vi "AlliGator Shot Noise Influence on Average Lifetime.vi"() -> ()   [LabVIEW 2021, in "AlliGator Shot Noise Influence on Average Lifetime.lvlib"]
doc: "Main window of the Shot Noise Influence on Average Lifetime tool."
uses:
  AlliGator Shot Noise Influence on Average Lifetime.lvlib
  AlliGator Statistics Simulation Parameters.ctl
  AlliGator Phasor Simulation Parameters.ctl
  Arrays/Array Statistics.ctl
  Graphs/XY Graph/XY Graph Event.ctl
  <vilib>/Utility/miscctls.llb/LVPoint32TypeDef.ctl
  1e2fc33e-f2e1-4865-bd35-b782600da79c.vi
  ffbda573-fdee-4728-9e4a-091745fb94a5.vi
  20485d49-49ee-422f-9a66-761cdf75a503.vi
  AlliGator Abort.vi
  GUI/GUI.lvlib
  Notebook/Notebook.lvlib
  Error/Error.lvlib
  AlliGator Globals, Variables & Constants.lvlib
  Graphs/XY Graph/XY Graph Add-Ons.lvlib
  Arrays/Arrays.lvlib
panel:
  in  "Random Seed":i32=1000
  in  "SDV Histogram Percentiles":dbl[](array[numeric])=[1.0, 99.0]
  in  "Lifetime Histogram Percentiles":dbl[](array[numeric])=[1.0, 99.0]
  out "Message":string caption="Output (see Notebook)"
  in  "Histogram Bin Size (SDV)":dbl[unit]=1.0000000000000002e-12
  out "AlliGator Approach SDVs":T1 {"Min" format="%#_4g"; "Max" format="%#_4g"; "Mean" format="%#_4g"; "Standard Deviation" format="%#_4g"}
  out "AlliGator Approach":T1 {"Min" format="%#_4g"; "Max" format="%#_4g"; "Mean" format="%#_4g"; "Standard Deviation" format="%#_4g"}
  out "Pure Poisson":T1 {"Min" format="%#_4g"; "Max" format="%#_4g"; "Mean" format="%#_4g"; "Standard Deviation" format="%#_4g"}
  in  "Histogram Bin Size (Lifetime)":dbl[unit]=1.0000000000000001e-11
  in  "Phasor Parameters":T2={"tau 1"=3e-10, "tau 2"=3.0000000000000004e-09, "f1"=0.5, "Frequency"=80000000.0}
  in  "Simulation Parameters":T3={"# Photons"=100, "# Replicas (M)"=1000, "# Simulations (N)"=1000, "Decay Bin Size"=1.0000000000000002e-10}
  in  "Run Simulation":bool
  out "Histograms":cluster{"Axis":dbl[], "Histogram":dbl[]}[](graph)
  in  "Animated Busy Icon":bool=TRUE
  in  "Abort":bool
  out "Progress Bar":dbl(slide) scale=0.0..100.0
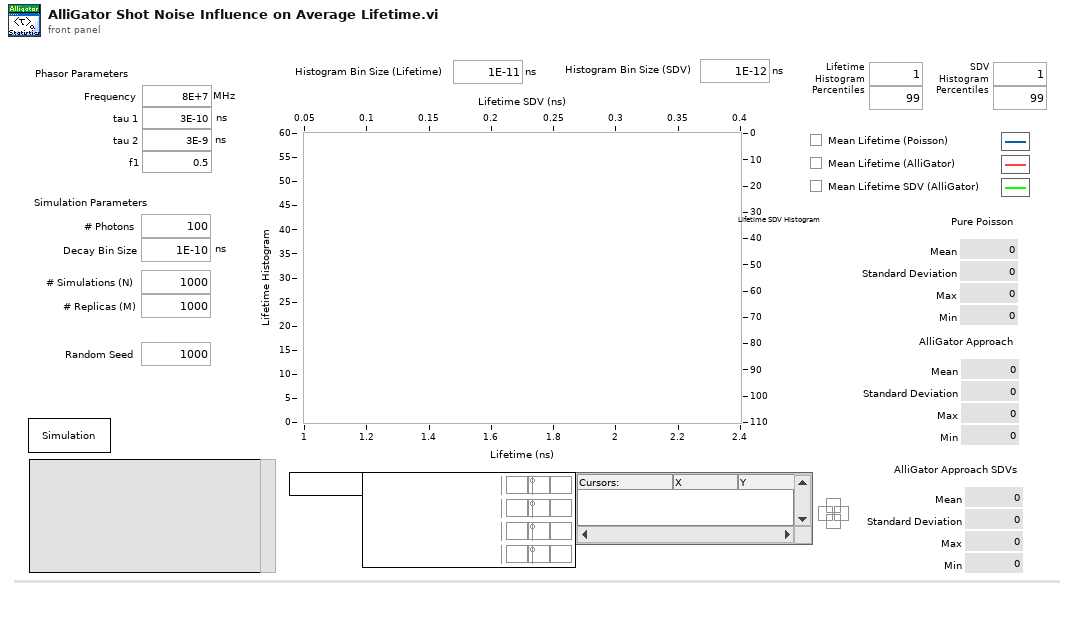
[diagram p1: front panel]
types:
  T1 = typedef "Arrays.lvlib/Array Statistics.ctl" = cluster{"Mean":dbl, "Standard Deviation":dbl, "Max":dbl, "Min":dbl}
  T2 = typedef "AlliGator Shot Noise Influence on Average Lifetime.lvlib/AlliGator Phasor Simulation Parameters.ctl" = cluster{"tau 1":dbl[unit], "tau 2":dbl[unit], "f1":dbl, "Frequency":dbl[unit]}
  T3 = typedef "AlliGator Shot Noise Influence on Average Lifetime.lvlib/AlliGator Statistics Simulation Parameters.ctl" = cluster{"# Photons":i32, "# Replicas (M)":i32, "# Simulations (N)":i32, "Decay Bin Size":dbl[unit]}
  T4 = typedef "XY Graph Add-Ons.lvlib/XY Graph Event.ctl" = cluster{"Item Tag":string, "XY Graph Refnum":refnum<vi>, "Coords":T5, "Item Path":string}
  T5 = typedef "LVPoint32TypeDef.ctl" = cluster{"Horizontal":i32, "Vertical":i32}
  T6 = typedef "AlliGator Progress Bar Q Element.ctl" = cluster{"Action":string, "Value":dbl}
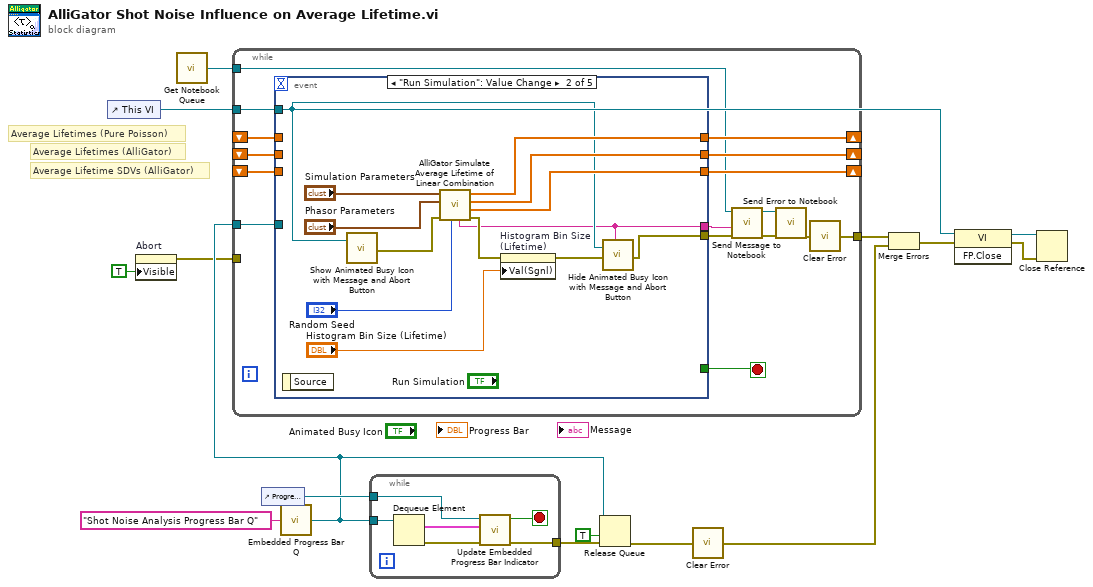
[diagram p0: block diagram]
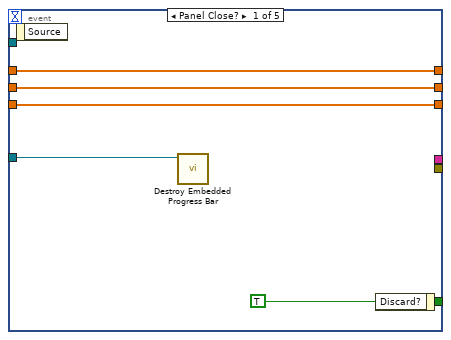
[diagram p2: hidden frame]
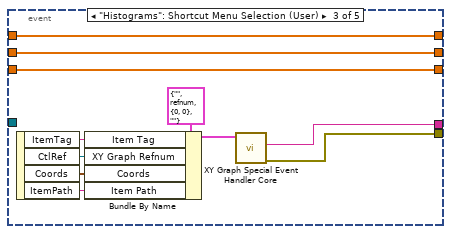
[diagram p3: hidden frame]
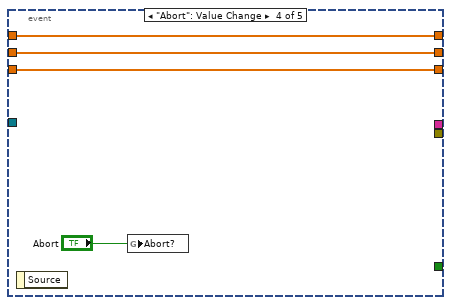
[diagram p4: hidden frame]
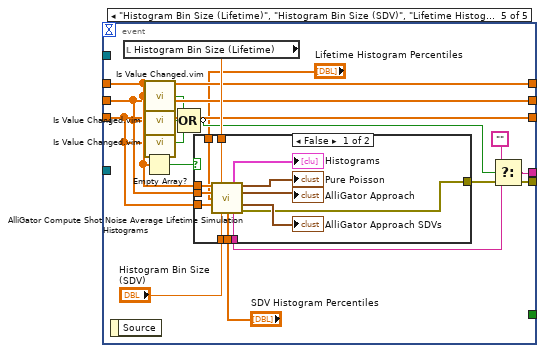
[diagram p5: hidden frame]
diagram:
  # "Average Lifetime SDVs (AlliGator)"
  # "Average Lifetimes (AlliGator)"
  # "Average Lifetimes (Pure Poisson)"
  n1 = control-ref of="This VI"() -> (w2:refnum<vi>)
  n2 = property on="Abort" class="Bool"("Visible"=TRUE) -> (error out=w3:errorcluster)  [unwired: 2 in, 1 out]
  n3 = call "Get Notebook Queue.vi"() -> ("Notebook Queue"=w10:refnum<queue>)  [unwired: 9 in]
  n4 = control-ref of="Progress Bar"() -> (w14:refnum<vi>)
  n5 = call "Embedded Progress Bar Q.vi"("Progress Bar Queue Name"="Shot Noise Analysis Progress Bar Q") -> ("Progress Bar Queue"=w11:refnum<queue>)  [unwired: 6 in]
  n6 = while {
    shift-right: [w30] -> _
    shift-left: _ -> [w27]
    shift-right: [w29] -> _
    shift-left: _ -> [w26]
    shift-right: [w28] -> _
    shift-left: _ -> [w25]
    tunnel: w11 -> [w24]
    tunnel: w10 -> [w23]
    tunnel: [w17] -> w9
    tunnel: w3 -> [_]
    tunnel: w2 -> [w16]
    stop <- w31 stop-if-true
    n7 = event shown="[1] \"Run Simulation\": Value Change" {
      selector: _ -> [_ _ _ _ _]
      dyn-events: _ -> [_ _ _ _ _]
      timeout: _ -> [_ _ _ _ _]
      tunnel: [w36 _ _ _ _] -> w31
      tunnel: [w35 w47 w60 w64 w76] -> w30
      tunnel: [w34 w46 w59 w63 w75] -> w29
      tunnel: [w33 w45 w58 w62 w74] -> w28
      tunnel: w27 -> [w35 _ w60 w64 w76]
      tunnel: w26 -> [w34 _ w59 w63 w75]
      tunnel: w25 -> [w33 _ w58 w62 w74]
      tunnel: w24 -> [w32 _ _ _ _]
      tunnel: [_ w38 w51 _ w68] -> w22
      tunnel: [_ w40 w50 _ w78] -> w18
      tunnel: w16 -> [_ w39 _ _ _]
      event Panel Close? {
        w36 = TRUE ("Discard?")
        n8 = event-data() -> ()  [unwired: 1 in, 1 out]
        n9 = call "Destroy Embedded Progress Bar.vi"("Progress Bar Queue in"=w32) -> ()  [unwired: 10 in, 1 out]
        n10 = event-data("Discard?"=w36) -> ()  [unwired: 1 in, 1 out]
      }
      event "Run Simulation": Value Change {
        n11 = event-data() -> ()  [unwired: 1 in, 1 out]
        n12 = call "Show Animated Busy Icon with Message and Abort Button.vi"("Target VI reference"=w39) -> ("Error Out"=w42:errorcluster)  [unwired: 18 in]
        n13 = call "AlliGator Simulate Average Lifetime of Linear Combination.vi"("seed"="Random Seed", "Error In"=w42, "Phasor Parameters"="Phasor Parameters", "Simulation Parameters"="Simulation Parameters") -> ("Error Out"=w43:errorcluster, "Average Lifetimes SDV (AlliGator)"=w45:dbl[], "Average Lifetimes (AlliGator)"=w46:dbl[], "Average Lifetimes (Pure Poisson)"=w47:dbl[], "Message"=w38:string)  [unwired: 3 in]
        n14 = property on="Histogram Bin Size (Lifetime)" class="DigNum (strict)"(error in=w43, "Val(Sgnl)"="Histogram Bin Size (Lifetime)") -> (error out=w41:errorcluster)  [unwired: 1 in, 1 out]
        n15 = call "Hide Animated Busy Icon with Message and Abort Button.vi"("Message"=w38, "Target VI reference"=w39, "Error In"=w41) -> ("Error Out"=w40:errorcluster)  [unwired: 16 in]
      }
      event "Histograms": Shortcut Menu Selection (User) {
        n16 = event-data() -> ("ItemTag"=w56:string, "CtlRef"=w55:refnum<vi>, "Coords"=w54:T5, "ItemPath"=w53:string)  [unwired: 1 in]
        n17 = Bundle By Name(cluster=T4 {"Item Tag"="", "XY Graph Refnum"=refnum, "Coords"={"Horizontal"=0, "Vertical"=0}, "Item Path"=""} ("XY Graph Event"), "Item Tag"=w56, "XY Graph Refnum"=w55, "Coords"=w54, "Item Path"=w53) -> (w52:T4)
        n18 = call "XY Graph Special Event Handler Core.vi"("XY Graph Event"=w52) -> ("error out"=w50:errorcluster, "Message"=w51:string)  [unwired: 6 in, 3 out]
      }
      event "Abort": Value Change {
        n19 = event-data() -> ()  [unwired: 1 in, 1 out]
        n20 = global write "AlliGator Abort.vi" "Abort?"("Abort") -> ()
      }
      event "Histogram Bin Size (Lifetime)", "Histogram Bin Size (SDV)", "Lifetime Histogram Percentiles", "SDV Histogram Percentiles": Value Change {
        n21 = event-data() -> ()  [unwired: 1 in, 1 out]
        n22 = local read "Histogram Bin Size (Lifetime)"() -> (w80:dbl[unit])
        n23 = Empty Array?(array=w76) -> (empty?=w77:bool)
        n24 = call "Is Value Changed.vim"("value"=w76) -> ("changed or first call?"=w73:bool)
        n25 = call "Is Value Changed.vim"("value"=w75) -> ("changed or first call?"=w72:bool)
        n26 = call "Is Value Changed.vim"("value"=w74) -> ("changed or first call?"=w71:bool)
        n27 = Compound Arithmetic op=OR(w73, w72, w71) -> (invert w70:bool)
        n28 = case shown="False" w77 {
          tunnel: w80 -> [w93 _]
          tunnel: w75 -> [w92 _]
          tunnel: w74 -> [w91 _]
          tunnel: w76 -> [w90 _]
          tunnel: "Histogram Bin Size (SDV)" -> [w89 _]
          tunnel: [w84 _] -> w69
          tunnel: [w83 _] -> w78
          tunnel: "Lifetime Histogram Percentiles" -> [w82 _]
          tunnel: "SDV Histogram Percentiles" -> [w81 _]
          frame False {
            n29 = call "AlliGator Compute Shot Noise Average Lifetime Simulation Histograms.vi"("Average Lifetimes (Pure Poisson)"=w90, "Histogram Bin Size"=w93, "Average Lifetimes (AlliGator)"=w92, "Lifetime Histo Percentiles"=w82, "Average Lifetime SDVs (AlliGator)"=w91, "Histogram Bin Size (SDV)"=w89, "SDV Histo Percentiles"=w81) -> ("Histograms"=→"Histograms":cluster{"Axis":dbl[], "Histogram":dbl[]}[], "Array Statistic (Pure Poisson)"=→"Pure Poisson":T1, "Array Statistics (AlliGator)"=→"AlliGator Approach":T1, "Array Statistics (AlliGator SDVs)"=→"AlliGator Approach SDVs":T1, "Message"=w84:string, "Error Out"=w83:errorcluster)  [unwired: 3 in]
          }
          frame True {
          }
        }
        n30 = Select(t="", s=w70, f=w69) -> (s? t:f=w68:string)
      }
    }
    n31 = call "Send Message to Notebook.vi"("Error In"=w18, "Message"=w22, "Notebook Queue"=w23) -> ("Error Out"=w20:errorcluster, "Notebook Queue"=w21:refnum<queue>)  [unwired: 5 in]
    n32 = call "Send Error to Notebook.vi"("error in (no error)"=w20, "Notebook Q"=w21) -> ("Error Out"=w19:errorcluster)  [unwired: 9 in]
    n33 = call "Clear Error.vi"("Error In"=w19) -> ("no Error Out"=w17:errorcluster)  [unwired: 8 in]
  }
  n34 = while {
    tunnel: w11 -> [w99]
    tunnel: w14 -> [w97]
    tunnel: [w94] -> w13
    stop <- w95 stop-if-true
    n35 = Dequeue Element(queue=w99) -> (element=w98:T6, error out=w96:errorcluster)  [unwired: 2 in, 2 out]
    n36 = call "Update Embedded Progress Bar Indicator.vi"("Error In"=w96, "Progress Bar Event"=w98, "Progress Bar Refnum"=w97) -> ("Error Out"=w94:errorcluster, "Quit?"=w95:bool)  [unwired: 7 in]
  }
  n37 = Release Queue(queue=w11, force destroy? (F)=TRUE, error in (no error)=w13) -> (error out=w8:errorcluster)  [unwired: 2 out]
  n38 = call "Clear Error.vi"("Error In"=w8) -> ("no Error Out"=w1:errorcluster)  [unwired: 8 in]
  n39 = Merge Errors(w9, w1) -> (w7:errorcluster)
  n40 = invoke class="VI" method="FP.Close"(reference=w2, error in=w7) -> (reference out=w6:refnum<vi>, error out=w5:errorcluster)  [unwired: 1 in, 1 out]
  n41 = Close Reference(reference=w6, error in (no error)=w5) -> ()  [unwired: 1 out]
